vi "FormatData.vi"(11 "Raw data":u64[](array[numeric])) -> (3 "Scaled":dbl[][](array[numeric]))   [LabVIEW 2025, in "FpgaRefx410.lvclass"]
uses:
  FpgaRefx410.lvclass
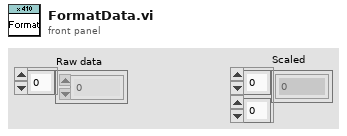
[diagram p1: front panel]
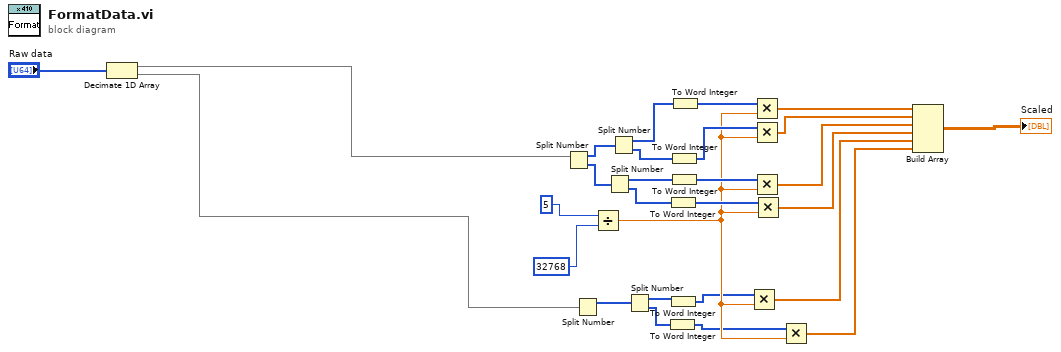
[diagram p0: block diagram]
diagram:
  n1 = Decimate 1D Array("Raw data") -> (w4:u64[], w3:u64[])
  n2 = Split Number(x=w4) -> (hi(x)=w25:u32[], lo(x)=w21:u32[])
  n3 = Split Number(x=w3) -> (hi(x)=w10:u32[])  [unwired: 1 out]
  n4 = Divide(x=5, y=32768) -> (x/y=w9:dbl)
  n5 = Split Number(x=w21) -> (hi(x)=w23:u16[], lo(x)=w24:u16[])
  n6 = Split Number(x=w25) -> (hi(x)=w26:u16[], lo(x)=w22:u16[])
  n7 = Split Number(x=w10) -> (hi(x)=w8:u16[], lo(x)=w7:u16[])
  n8 = To Word Integer(number=w7) -> (16bit integer=w5:i16[])
  n9 = To Word Integer(number=w24) -> (16bit integer=w16:i16[])
  n10 = To Word Integer(number=w8) -> (16bit integer=w6:i16[])
  n11 = To Word Integer(number=w22) -> (16bit integer=w18:i16[])
  n12 = To Word Integer(number=w23) -> (16bit integer=w17:i16[])
  n13 = To Word Integer(number=w26) -> (16bit integer=w20:i16[])
  n14 = Multiply(x=w6, y=w9) -> (x*y=w11:dbl[])
  n15 = Multiply(x=w20, y=w9) -> (x*y=w19:dbl[])
  n16 = Multiply(x=w18, y=w9) -> (x*y=w15:dbl[])
  n17 = Multiply(x=w17, y=w9) -> (x*y=w14:dbl[])
  n18 = Multiply(x=w16, y=w9) -> (x*y=w13:dbl[])
  n19 = Multiply(x=w5, y=w9) -> (x*y=w12:dbl[])
  n20 = Build Array(w19, w15, w14, w13, w11, w12) -> (→"Scaled":dbl[][])
